vi "ProdaNG.All.vi"() -> ()   [LabVIEW 2016]
uses:
  LowLevel/ProdaNG.Global.vi
panel:
  in  "Changelog":string="Wabco ProdaNG LabVIEW interface\nTest & Measurement Solutions\nMaciej Szupienko\n---------------------------------------------------------------------\n\nv2015.10.29.1\n- prodllNG.dll v2015.07.29.1\n- get rid of wrapper dll"
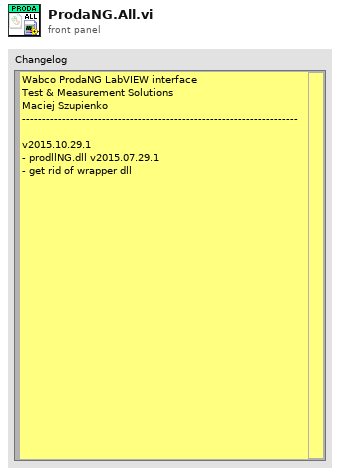
[diagram p1: front panel]
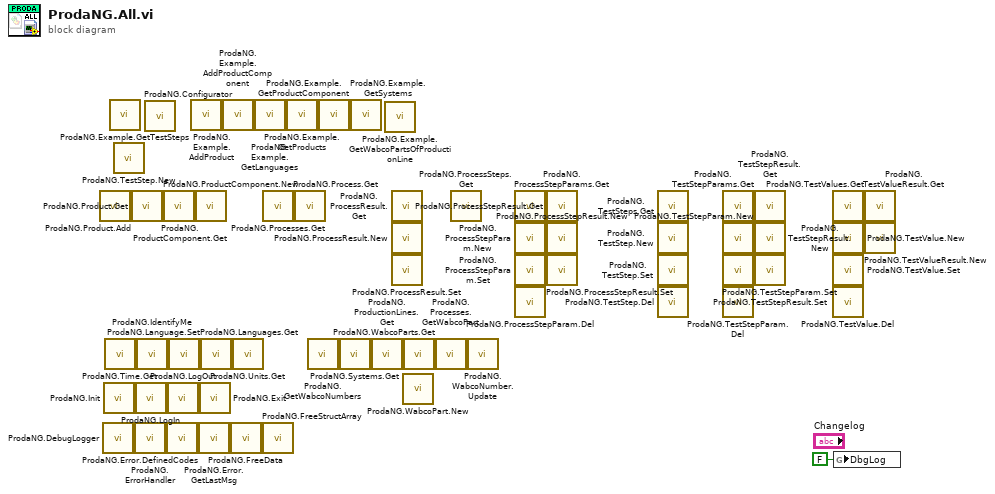
[diagram p0: block diagram]
diagram:
  n1 = call "ProdaNG.Product.Add.vi"() -> ()  [unwired: 9 in, 3 out]
  n2 = call "ProdaNG.DebugLogger.vi"() -> ()  [unwired: 11 in, 1 out]
  n3 = call "ProdaNG.Init.vi"() -> ()  [unwired: 11 in, 1 out]
  n4 = call "ProdaNG.Time.Get.vi"() -> ()  [unwired: 7 in, 4 out]
  n5 = call "ProdaNG.Example.GetTestSteps.vi"() -> ()  [unwired: 12 in]
  n6 = call "ProdaNG.TestStep.New.vi"() -> ()  [unwired: 9 in, 3 out]
  n7 = call "ProdaNG.Product.Get.vi"() -> ()  [unwired: 8 in, 4 out]
  n8 = call "ProdaNG.ErrorHandler.vi"() -> ()  [unwired: 11 in, 1 out]
  n9 = call "ProdaNG.LogIn.vi"() -> ()  [unwired: 9 in, 3 out]
  n10 = call "ProdaNG.IdentifyMe.vi"() -> ()  [unwired: 9 in, 3 out]
  n11 = call "ProdaNG.Configurator.vi"() -> ()  [unwired: 12 in]
  n12 = call "ProdaNG.ProductComponent.New.vi"() -> ()  [unwired: 10 in, 2 out]
  n13 = call "ProdaNG.Error.DefinedCodes.vi"() -> ()  [unwired: 5 in, 3 out]
  n14 = call "ProdaNG.LogOut.vi"() -> ()  [unwired: 11 in, 1 out]
  n15 = call "ProdaNG.Language.Set.vi"() -> ()  [unwired: 10 in, 2 out]
  n16 = call "ProdaNG.Example.AddProduct.vi"() -> ()  [unwired: 12 in]
  n17 = call "ProdaNG.ProductComponent.Get.vi"() -> ()  [unwired: 9 in, 3 out]
  n18 = call "ProdaNG.Error.GetLastMsg.vi"() -> ()  [unwired: 10 in, 2 out]
  n19 = call "ProdaNG.Exit.vi"() -> ()  [unwired: 11 in, 1 out]
  n20 = call "ProdaNG.Languages.Get.vi"() -> ()  [unwired: 9 in, 3 out]
  n21 = call "ProdaNG.Example.AddProductComponent.vi"() -> ()  [unwired: 12 in]
  n22 = call "ProdaNG.FreeData.vi"() -> ()  [unwired: 11 in, 1 out]
  n23 = call "ProdaNG.Units.Get.vi"() -> ()  [unwired: 8 in, 4 out]
  n24 = call "ProdaNG.Example.GetLanguages.vi"() -> ()  [unwired: 12 in]
  n25 = call "ProdaNG.Processes.Get.vi"() -> ()  [unwired: 9 in, 3 out]
  n26 = call "ProdaNG.FreeStructArray.vi"() -> ()  [unwired: 11 in, 1 out]
  n27 = call "ProdaNG.Example.GetProducts.vi"() -> ()  [unwired: 12 in]
  n28 = call "ProdaNG.Process.Get.vi"() -> ()  [unwired: 8 in, 4 out]
  n29 = call "ProdaNG.GetWabcoNumbers.vi"() -> ()  [unwired: 8 in, 4 out]
  n30 = call "ProdaNG.Example.GetProductComponent.vi"() -> ()  [unwired: 12 in]
  n31 = call "ProdaNG.Systems.Get.vi"() -> ()  [unwired: 9 in, 3 out]
  n32 = call "ProdaNG.Example.GetSystems.vi"() -> ()  [unwired: 12 in]
  n33 = call "ProdaNG.ProductionLines.Get.vi"() -> ()  [unwired: 9 in, 3 out]
  n34 = call "ProdaNG.Example.GetWabcoPartsOfProductionLine.vi"() -> ()  [unwired: 12 in]
  n35 = call "ProdaNG.ProcessResult.Get.vi"() -> ()  [unwired: 8 in, 4 out]
  n36 = call "ProdaNG.ProcessResult.New.vi"() -> ()  [unwired: 9 in, 3 out]
  n37 = call "ProdaNG.ProcessResult.Set.vi"() -> ()  [unwired: 10 in, 2 out]
  n38 = call "ProdaNG.WabcoPart.New.vi"() -> ()  [unwired: 10 in, 2 out]
  n39 = call "ProdaNG.WabcoParts.Get.vi"() -> ()  [unwired: 9 in, 3 out]
  n40 = call "ProdaNG.Processes.GetWabcoPart.vi"() -> ()  [unwired: 9 in, 3 out]
  n41 = call "ProdaNG.ProcessSteps.Get.vi"() -> ()  [unwired: 9 in, 3 out]
  n42 = call "ProdaNG.WabcoNumber.Update.vi"() -> ()  [unwired: 10 in, 2 out]
  n43 = call "ProdaNG.ProcessStepParams.Get.vi"() -> ()  [unwired: 9 in, 3 out]
  n44 = call "ProdaNG.ProcessStepParam.New.vi"() -> ()  [unwired: 9 in, 3 out]
  n45 = call "ProdaNG.ProcessStepParam.Set.vi"() -> ()  [unwired: 9 in, 3 out]
  n46 = call "ProdaNG.ProcessStepParam.Del.vi"() -> ()  [unwired: 10 in, 2 out]
  n47 = call "ProdaNG.ProcessStepResult.Get.vi"() -> ()  [unwired: 8 in, 4 out]
  n48 = call "ProdaNG.ProcessStepResult.New.vi"() -> ()  [unwired: 9 in, 3 out]
  n49 = call "ProdaNG.ProcessStepResult.Set.vi"() -> ()  [unwired: 10 in, 2 out]
  n50 = call "ProdaNG.TestSteps.Get.vi"() -> ()  [unwired: 9 in, 3 out]
  n51 = call "ProdaNG.TestStep.New.vi"() -> ()  [unwired: 9 in, 3 out]
  n52 = call "ProdaNG.TestStep.Set.vi"() -> ()  [unwired: 9 in, 3 out]
  n53 = call "ProdaNG.TestStep.Del.vi"() -> ()  [unwired: 10 in, 2 out]
  n54 = call "ProdaNG.TestStepParams.Get.vi"() -> ()  [unwired: 9 in, 3 out]
  n55 = call "ProdaNG.TestStepParam.New.vi"() -> ()  [unwired: 9 in, 3 out]
  n56 = call "ProdaNG.TestStepParam.Set.vi"() -> ()  [unwired: 9 in, 3 out]
  n57 = call "ProdaNG.TestStepParam.Del.vi"() -> ()  [unwired: 10 in, 2 out]
  n58 = call "ProdaNG.TestStepResult.Get.vi"() -> ()  [unwired: 8 in, 4 out]
  n59 = call "ProdaNG.TestStepResult.New.vi"() -> ()  [unwired: 9 in, 3 out]
  n60 = call "ProdaNG.TestStepResult.Set.vi"() -> ()  [unwired: 10 in, 2 out]
  n61 = call "ProdaNG.TestValues.Get.vi"() -> ()  [unwired: 9 in, 3 out]
  n62 = call "ProdaNG.TestValue.New.vi"() -> ()  [unwired: 9 in, 3 out]
  n63 = call "ProdaNG.TestValue.Set.vi"() -> ()  [unwired: 9 in, 3 out]
  n64 = call "ProdaNG.TestValue.Del.vi"() -> ()  [unwired: 10 in, 2 out]
  n65 = global write "ProdaNG.Global.vi" "DbgLog"(FALSE ("DbgLog")) -> ()
  n66 = call "ProdaNG.TestValueResult.Get.vi"() -> ()  [unwired: 9 in, 3 out]
  n67 = call "ProdaNG.TestValueResult.New.vi"() -> ()  [unwired: 10 in, 2 out]
